vi "TestPG.vi"() -> ()   [LabVIEW 2018]
uses:
  Quantum Composers 9000 Series.lvlib
panel:
  out "Pulse Generator Error":errorcluster
  in  "Cycle time\n(ms)":i32=3 min=0 step=1
  in  "MODE":u16(ring) items=["Normal", "DIF"]
  in  "BIN":u16(ring)=2 items=["1x1", "2x2", "4x4"]
  in  "# Frames":i32=1000 min=0 step=1
  in  "On CCD Acc.":i32=3 min=0 step=1
  in  "stop":bool
  in  "RUN/STOP":bool
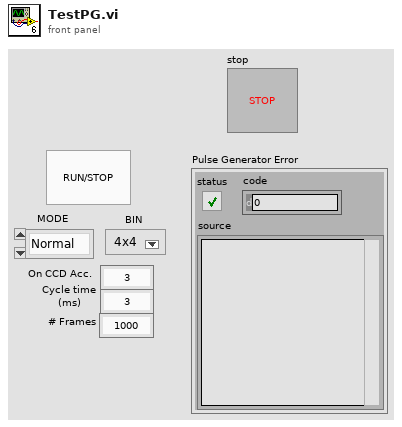
[diagram p1: front panel]
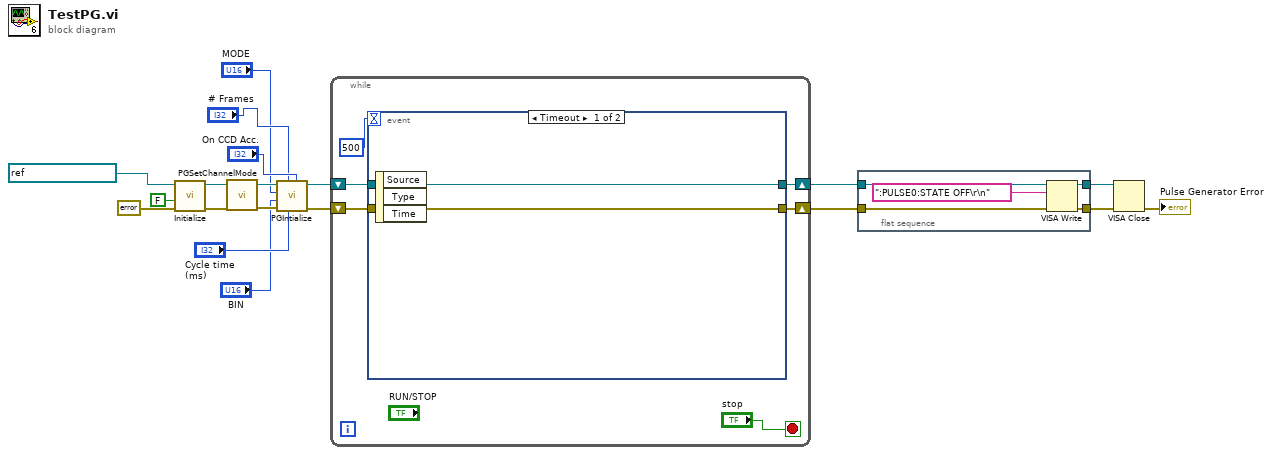
[diagram p0: block diagram]
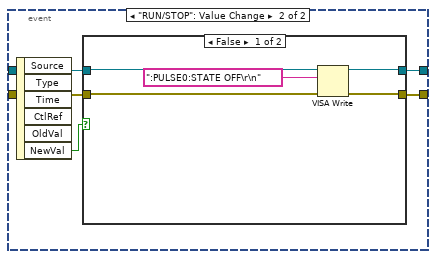
[diagram p2: hidden frame]
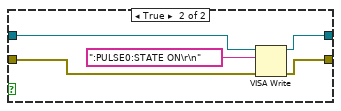
[diagram p3: hidden frame]
diagram:
  n1 = call "Initialize.vi"("error in (no error)"=errorcluster {"status"=FALSE, "code"=0, "source"=""}, "Reset? (T: Yes)"=FALSE, "VISA resource name"=refnum<visa-resource-name> "PulseGenerator" ("Pulse generater (COM3)")) -> ("error out"=w17:errorcluster, "VISA resource name out"=w16:refnum<visa-resource-name>)  [unwired: 7 in]
  n2 = call "PGSetChannelMode.vi"("error in"=w17, "VISA resource name"=w16) -> ("error out"=w15:errorcluster, "VISA resource name out"=w13:refnum<visa-resource-name>)  [unwired: 8 in]
  n3 = call "PGIntialize.vi"("On CCD Accumulations"="On CCD Acc.", "Cycle time\n(ms)"="Cycle time\n(ms)", "Number of Frames"="# Frames", "error in"=w15, "BIN"="BIN", "MODE"="MODE", "VISA resource name"=w13) -> ("error out"=w14:errorcluster, "VISA resource name out"=w12:refnum<visa-resource-name>)  [unwired: 3 in]
  n4 = while {
    shift-right: [w21] -> w3
    shift-left: w14 -> [w25]
    shift-right: [w22] -> w2
    shift-left: w12 -> [w24]
    stop <- "stop" stop-if-true
    n5 = event shown="[0] Timeout" {
      selector: _ -> [_ _]
      dyn-events: _ -> [_ _]
      timeout: 500 ("Numeric") -> [_ _]
      tunnel: w25 -> [w26 w31]
      tunnel: w24 -> [w27 w30]
      tunnel: [w27 w29] -> w22
      tunnel: [w26 w28] -> w21
      event Timeout {
        n6 = event-data() -> ()  [unwired: 1 in, 3 out]
      }
      event "RUN/STOP": Value Change {
        n7 = event-data() -> ("NewVal"=w32:bool)  [unwired: 1 in, 5 out]
        n8 = case shown="False" w32 {
          tunnel: w31 -> [w35 w41]
          tunnel: w30 -> [w36 w40]
          tunnel: [w33 w39] -> w29
          tunnel: [w34 w38] -> w28
          frame False {
            n9 = VISA Write(VISA resource name=w36, write buffer=":PULSE0:STATE OFF\r\n" ("format string"), error in (no error)=w35) -> (VISA resource name out=w33:refnum<visa-resource-name>, error out=w34:errorcluster)  [unwired: 1 out]
          }
          frame True {
            n10 = VISA Write(VISA resource name=w40, write buffer=":PULSE0:STATE ON\r\n" ("format string"), error in (no error)=w41) -> (VISA resource name out=w39:refnum<visa-resource-name>, error out=w38:errorcluster)  [unwired: 1 out]
          }
        }
      }
    }
  }
  n11 = flat-sequence {
    tunnel: [w46] -> w4
    tunnel: [w45] -> w5
    tunnel: w2 -> [w44]
    tunnel: w3 -> [w43]
    frame #0 {
      n12 = VISA Write(VISA resource name=w44, write buffer=":PULSE0:STATE OFF\r\n" ("format string"), error in (no error)=w43) -> (VISA resource name out=w45:refnum<visa-resource-name>, error out=w46:errorcluster)  [unwired: 1 out]
    }
  }
  n13 = VISA Close(VISA resource name=w5, error in (no error)=w4) -> (error out=→"Pulse Generator Error":errorcluster)
